vi "PGSQL test.vi"() -> ()   [LabVIEW 2016, in "instrument.PPMS.lvclass"]
uses:
  instrument.PPMS.lvclass
  Typedefs/PPMS.getAll--cluster.ctl
panel:
  out "string":string
  out "error out":errorcluster
  in  "error in (no error)":errorcluster
  out "VCluster 2":variant
  out "VCluster":variant
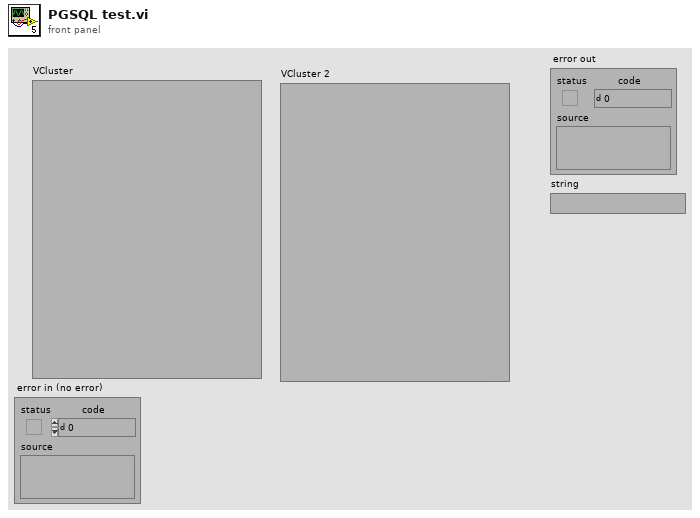
[diagram p1: front panel]
types:
  T1 = typedef "instrument.PPMS.lvclass/PPMS.getAll--cluster.ctl" = cluster{"Helium Level (%)":dbl, "Temperature (K)":dbl, "Temperature Status":string, "Magnetic Field (T)":dbl, "Magnet Status":string, "Position (°)":dbl}
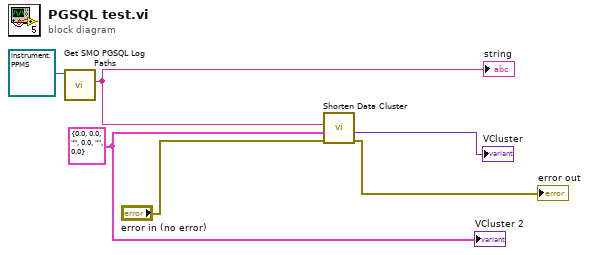
[diagram p0: block diagram]
diagram:
  w4 = T1 {"Helium Level (%)"=0.0, "Temperature (K)"=0.0, "Temperature Status"="", "Magnetic Field (T)"=0.0, "Magnet Status"="", "Position (°)"=0.0} ("getAll")
  n1 = call-dynamic "Get SMO PGSQL Log Paths.vi"("instrument.PPMS in"=refnum<class "instrument.PPMS.lvclass"> refnum) -> ("Paths"=w1:string)  [unwired: 8 in, 2 out]
  "string" <- w1
  n2 = call <userlib>:"Shorten Data Cluster.vi"("error in (no error)"="error in (no error)", "Variant"=w4, "Paths"=w1) -> ("error out"=→"error out":errorcluster, "VCluster"=→"VCluster":variant)  [unwired: 5 in, 1 out]
  "VCluster 2" <- w4
